vi "Initialize Stage Controller.vi"(8 "error in (no error)":errorcluster, 11 "Application in":refnum<class "Application.lvclass">) -> (0 "error out":errorcluster, 3 "Application out":refnum<class "Application.lvclass">)   [LabVIEW 2015, in "Application.lvlib" / "Application.lvclass"]
uses:
  Application.lvclass
  Hardware/Stage Controller/Stage Controller.lvclass
  Application.lvclass/Application.ctl
  <vilib>/ActorFramework/Actor/Actor.lvclass
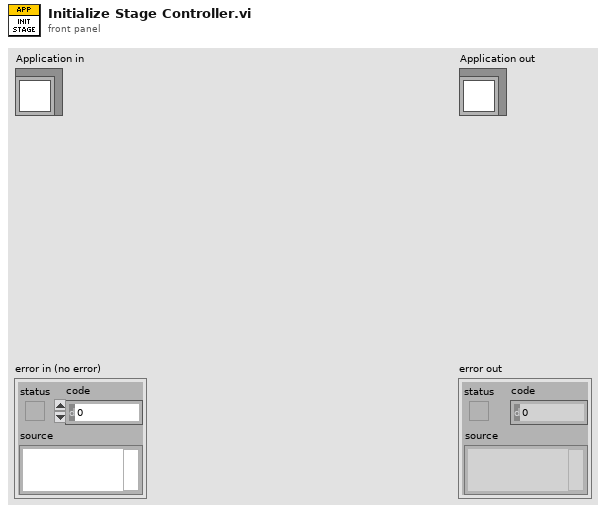
[diagram p1: front panel]
types:
  T1 = typedef "Stage Configuration.ctl" = cluster{"Serial Port":refnum<visa-resource-name>, "Forward Step (mm)":dbl, "Lane Length (mm)":dbl, "Lane Separation (mm)":dbl}
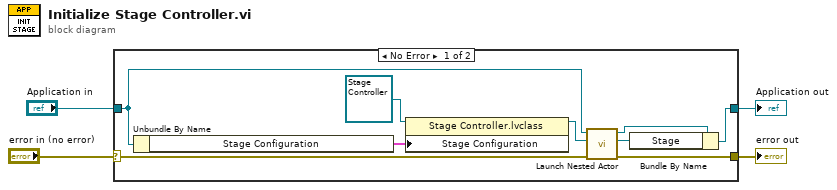
[diagram p0: block diagram]
diagram:
  n1 = case shown="No Error" "error in (no error)" {
    selector: "error in (no error)" -> [w5 w15]
    tunnel: [w11 w15] -> w3
    tunnel: [w12 w14] -> w1
    tunnel: "Application in" -> [w7 w14]
    frame No Error {
      n2 = Unbundle By Name(w7) -> ("Stage Configuration"=w6:T1)
      n3 = property class="Stage Controller.lvclass"(reference=refnum<class "Stage Controller.lvclass"> refnum ("Stage Controller.lvlib:Stage Controller.lvclass"), "Stage Configuration"=w6) -> (reference out=w9:refnum<class "Stage Controller.lvclass">)  [unwired: 1 in, 1 out]
      n4 = call <vilib>:"Launch Nested Actor.vi"("error in (no error)"=w5, "Nested Actor"=w9, "Caller Actor in"=w7) -> ("error out"=w11:errorcluster, "Nested Actor's Enqueuer"=w13:refnum<class "Message Enqueuer.lvclass">, "Caller Actor out"=w8:refnum<class "Application.lvclass">)  [unwired: 6 in]
      n5 = Bundle By Name(cluster=w8, "Stage"=w13) -> (w12:refnum<class "Application.lvclass">)
    }
    frame Error {
    }
  }
  "error out" <- w3
  "Application out" <- w1
